vi "Panel Output Voltage Test.vi"(7 "Test Socket (0)":i32, 11 "DMM in":string) -> (0 "error out":errorcluster, 3 "Voltage":dbl)   [LabVIEW 2025]
doc: "Measures the voltage produced by the solar panel after setting the ambient lighting and temperature conditions."
uses:
  Program Files (x86)/National Instruments/LabVIEW 2024/Instr.lib/Driver Simulation/DMM/Signal Types.ctl
  Program Files (x86)/National Instruments/LabVIEW 2024/Instr.lib/Driver Simulation/DMM.lvlib
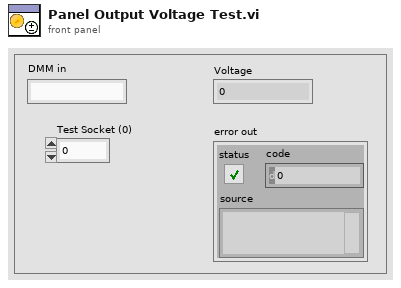
[diagram p1: front panel]
types:
  T1 = typedef "Driver Simulation.lvlib/DMM.lvlib/Signal Types.ctl" = enum16{"DC", "AC"}
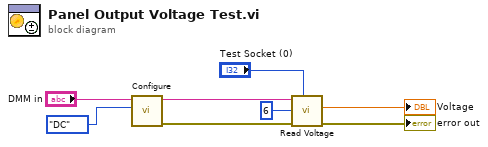
[diagram p0: block diagram]
diagram:
  n1 = call "Configure.vi"("Signal Type"=Signal_Types."DC", "DMM in"="DMM in") -> ("error out"=w8:errorcluster, "DMM out"=w6:string)  [unwired: 8 in]
  n2 = call "Read Voltage.vi"("Test Socket (0)"="Test Socket (0)", "error in (no error)"=w8, "Channel"=6, "DMM in"=w6) -> ("error out"=→"error out":errorcluster, "Voltage"=→"Voltage":dbl)  [unwired: 5 in, 1 out]
